vi "Actor Core.vi"(8 "error in":errorcluster, 11 "Test Executive Builder Dirty Dot View In":refnum<class "Test Executive Builder Dirty Dot View.lvclass">) -> (0 "error out":errorcluster, 3 "Actor out":refnum<class "Actor.lvclass">)   [LabVIEW 2017, in "Test Executive Builder Dirty Dot View.lvclass"]
doc: "(<B>Filename</B>: Actor Framework.lvlib:Actor.lvclass:Actor Core.vi)\n\nReceives messages to the actor, reacts to them, and initiates any error handling that may shut the actor down.\n\nDescendant classes may override this VI to append parallel tasks for the actor to complete while it handles messages. Overrides use the Call Parent Method node.\n\n<License>\nCopyright © 2017 Composed Systems, LLC | All rights reserved\nwww.composed.io\n\nAuthor: Ethan Stern <ethan.stern@composed.io>\n\nThis software is provided \"AS IS\" WITHOUT WARRANTIES, either express or implied, AND IS FOR EDUCATIONAL PURPOSES ONLY.\n</License>"
uses:
  Test Executive Builder Dirty Dot View.lvclass
  <vilib>/gpm_packages/@cs/mva-viewable/Source/IViewable/IViewable/IViewable.lvclass
  <vilib>/gpm_packages/@cs/mva-core/Source/IObserver/IObserver/IObserver.lvclass
  Test Executive Builder Dirty Dot View Messages/Update Dirty Dot Image Msg/Update Dirty Dot Image Msg.lvclass
  <vilib>/gpm_packages/@cs/mva-core/Source/SubscriptionPolicy/BasicSubscription/BasicSubscription.lvclass
  C:/Users/jonmc/Documents/Git/Test Executive Builder/gpm_packages/@cs/mva-core/Source/IMediator/ISubscriptionPolicy/ISubscriptionPolicy.lvclass
  C:/Users/jonmc/Documents/Git/Test Executive Builder/gpm_packages/@cs/transport/Source/Concrete/ActorMessageTransport/Notification Msg/Notification Msg.lvclass
  C:/Users/jonmc/Documents/Git/Test Executive Builder/gpm_packages/@cs/mva-core/Source/IObserver/IObserver/IObserver.lvclass
  <vilib>/ActorFramework/Actor/Actor.lvclass
panel:
  out "Dirty Dot":picture
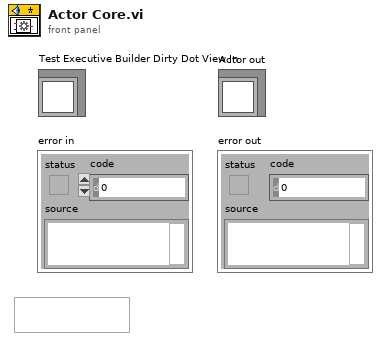
[diagram p1: front panel]
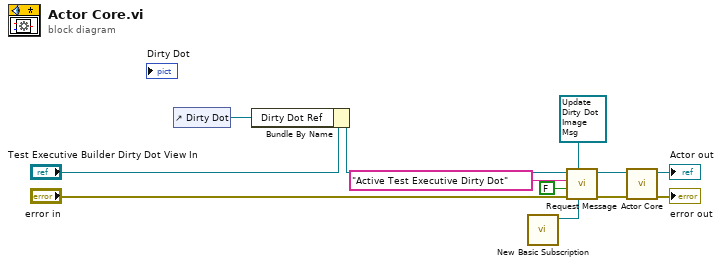
[diagram p0: block diagram]
diagram:
  n1 = control-ref of="Dirty Dot"() -> (w10:refnum<vi>)
  n2 = Bundle By Name(cluster="Test Executive Builder Dirty Dot View In", "Dirty Dot Ref"=w10) -> (w8:refnum<class "Test Executive Builder Dirty Dot View.lvclass">)
  n3 = call <vilib>:"New Basic Subscription.vi"() -> ("BasicSubscription Out"=w1:refnum<class "BasicSubscription.lvclass">)  [unwired: 11 in]
  n4 = call <vilib>:"Request Message.vi"("Configured SubscriptionPolicy"=w1, "Desired Notification Msg"=refnum<class "Update Dirty Dot Image Msg.lvclass"> refnum ("Update Dirty Dot Image Msg.lvclass"), "error in (no error)"="error in", "Data Type"=FALSE, "Datum Name"="Active Test Executive Dirty Dot", "IObserver in"=w8) -> ("error out"=w5:errorcluster, "IObserver out"=w7:refnum<class "Test Executive Builder Dirty Dot View.lvclass">)  [unwired: 3 in, 1 out]
  n5 = call-parent "Actor Core.vi"("error in"=w5, "IViewable In"=w7) -> ("error out"=→"error out":errorcluster, "Actor out"=→"Actor out":refnum<class "Actor.lvclass">)  [unwired: 8 in]
